vi "Device VI 1.2.vi"() -> ()   [LabVIEW 2017]
uses:
  <vilib>/Utility/error.llb/DialogType.ctl
  <vilib>/DAQmx/read.llb/DAQmx Read (Analog 1D Wfm NChan NSamp).vi
  <vilib>/DAQmx/create/channels.llb/DAQmx Create Channel (AI-Force-Bridge-Two-Point-Linear).vi
  <vilib>/DAQmx/configure/timing.llb/DAQmx Timing (Sample Clock).vi
  <vilib>/DAQmx/configure/trigger.llb/DAQmx Start Trigger (Digital Edge).vi
  <vilib>/DAQmx/configure/trigger.llb/DAQmx Start Trigger (Analog Edge).vi
  <vilib>/DAQmx/miscellaneous.llb/DAQmx Fill In Error Info.vi
  <resource>/objmgr/daqmx.rc
panel:
  in  "Filename":path=path "C:/Users/Julio/Desktop/Device Data/Test.xlsx"
  in  "Maximum Force":dbl=100.0
  in  "Minimum Force":dbl=-100.0
  in  "Units (Force)":i32(ring)=15875 items=["Newtons"=15875, "Pounds"=15876, "kgf"=15877, "From Custom Scale"=10065]
  in  "Trigger Type":T1(tab)
  in  "Digital Start Trigger Edge":i32(ring)=10280 caption="Edge" items=["Rising"=10280, "Falling"=10171]
  in  "Digital Start Trigger Source":tag="OnboardClock" caption="Source"
  in  "Digital Pause Trigger Pause When":i32(ring)=10192 caption="Pause When" items=["High"=10192, "Low"=10214]
  in  "Digital Pause Trigger Source":tag="/Dev1/PFI0" caption="Source"
  in  "Analog Start Trigger Level":dbl caption="Level" format="%0.2f"
  in  "Analog Start Trigger Hysteresis":dbl caption="Hysteresis" format="%.2f"
  in  "Analog Start Trigger Slope":i32(ring)=10280 caption="Slope" items=["Rising"=10280, "Falling"=10171]
  in  "Analog Start Trigger Source":string="APFI0" caption="Source"
  in  "Analog Pause Trigger Source":string="APFI0" caption="Source"
  in  "Analog Pause Trigger Pause When":i32(ring)=10093 caption="Pause When" items=["Above Level"=10093, "Below Level"=10107]
  in  "Analog Pause Trigger Level":dbl caption="Level" format="%.2f"
  in  "Bridge Information":T2={"Bridge Configuration"=10182, "Excitation Source"=10200, "Excitation Value"=2.5, "Nominal Resistance"=350.0} {"Excitation Source" items=["Internal"=10200, "External"=10167, "None"=10230]; "Bridge Configuration" items=["Full Bridge"=10182, "Half Bridge"=10187, "Quarter Bridge"=10270, "No Bridge"=10228]}
  in  "Physical Channel":tag="cDAQ2Mod1/ai0:cDAQ2Mod1/ai1"
  in  "Sample Rate":dbl=100.0
  in  "Samples per Loop":i32=100
  in  "Stop":bool
  out "Waveform Chart":waveform(dbl)[](graph)=[{"t0"=timestamp(3612197930.5365286 s since 1904-01-01), "dt"=0.01, "Y"=[-0.00735334478104631, -0.00735334478104631, -0.00735334478104631, -0.00735334478104631, -0.00735334478104631, -0.00735334478104631, -0.00735334478104631, -0.00735334478104631, -0.00735334478104631, -0.00735334478104631, -0.00735334478104631, -0.00735334478104631, -0.00735334478104631, -0.00735334478104631, -0.00735334478104631, -0.00735334478104631, -0.00735334478104631, -0.00735334478104631, -0.00735334478104631, -0.00735334478104631, -0.00735334478104631, -0.00735334478104631, -0.00735334478104631, -0.00735334478104631, -0.00735334478104631, -0.00735334478104631, -0.00735334478104631, -0.00735334478104631, -0.00735334478104631, -0.00735334478104631, -0.00735334478104631, -0.00735334478104631, -0.00735334478104631, -0.00735334478104631, -0.00735334478104631, -0.00735334478104631, -0.00735334478104631, -0.00735334478104631, -0.00735334478104631, -0.00735334478104631, -0.00735334478104631, -0.00735334478104631, -0.00735334478104631, -0.00735334478104631, -0.00735334478104631, -0.00735334478104631, -0.00735334478104631, -0.00735334478104631, -0.00735334478104631, -0.00735334478104631, -0.016674486052795045, -0.016674486052795045, -0.016674486052795045, -0.016674486052795045, -0.016674486052795045, -0.016674486052795045, -0.016674486052795045, -0.016674486052795045, -0.016674486052795045, -0.016674486052795045, -0.016674486052795045, -0.016674486052795045, -0.016674486052795045, -0.016674486052795045, -0.016674486052795045, -0.016674486052795045, -0.016674486052795045, -0.016674486052795045, -0.016674486052795045, -0.016674486052795045, -0.016674486052795045, -0.016674486052795045, -0.016674486052795045, -0.016674486052795045, -0.016674486052795045, -0.016674486052795045, -0.016674486052795045, -0.016674486052795045, -0.016674486052795045, -0.016674486052795045, -0.016674486052795045, -0.016674486052795045, -0.016674486052795045, -0.016674486052795045, -0.016674486052795045, -0.016674486052795045, -0.016674486052795045, -0.016674486052795045, -0.016674486052795045, -0.016674486052795045, -0.016674486052795045, -0.016674486052795045, -0.016674486052795045, -0.016674486052795045, -0.016674486052795045, -0.016674486052795045, -0.016674486052795045, -0.016674486052795045, -0.016674486052795045, -0.016674486052795045], "attributes"=variant("NI_ChannelName"=variant(string "cDAQ2Mod1/ai0"), "NI_UnitDescription"=variant(string "Newtons"))}, {"t0"=timestamp(3612197930.5365286 s since 1904-01-01), "dt"=0.01, "Y"=[0.0030034788542301913, 0.0030034788542301913, 0.0030034788542301913, 0.0030034788542301913, 0.0030034788542301913, 0.0030034788542301913, 0.0030034788542301913, 0.0030034788542301913, 0.0030034788542301913, 0.0030034788542301913, 0.0030034788542301913, 0.0030034788542301913, 0.0030034788542301913, 0.0030034788542301913, 0.0030034788542301913, 0.0030034788542301913, 0.0030034788542301913, 0.0030034788542301913, 0.0030034788542301913, 0.0030034788542301913, 0.0030034788542301913, 0.0030034788542301913, 0.0030034788542301913, 0.0030034788542301913, 0.0030034788542301913, 0.0030034788542301913, 0.0030034788542301913, 0.0030034788542301913, 0.0030034788542301913, 0.0030034788542301913, 0.0030034788542301913, 0.0030034788542301913, 0.0030034788542301913, 0.0030034788542301913, 0.0030034788542301913, 0.0030034788542301913, 0.0030034788542301913, 0.0030034788542301913, 0.0030034788542301913, 0.0030034788542301913, 0.0030034788542301913, 0.0030034788542301913, 0.0030034788542301913, 0.0030034788542301913, 0.0030034788542301913, 0.0030034788542301913, 0.0030034788542301913, 0.0030034788542301913, 0.0030034788542301913, 0.0030034788542301913, 0.00963184598080707, 0.00963184598080707, 0.00963184598080707, 0.00963184598080707, 0.00963184598080707, 0.00963184598080707, 0.00963184598080707, 0.00963184598080707, 0.00963184598080707, 0.00963184598080707, 0.00963184598080707, 0.00963184598080707, 0.00963184598080707, 0.00963184598080707, 0.00963184598080707, 0.00963184598080707, 0.00963184598080707, 0.00963184598080707, 0.00963184598080707, 0.00963184598080707, 0.00963184598080707, 0.00963184598080707, 0.00963184598080707, 0.00963184598080707, 0.00963184598080707, 0.00963184598080707, 0.00963184598080707, 0.00963184598080707, 0.00963184598080707, 0.00963184598080707, 0.00963184598080707, 0.00963184598080707, 0.00963184598080707, 0.00963184598080707, 0.00963184598080707, 0.00963184598080707, 0.00963184598080707, 0.00963184598080707, 0.00963184598080707, 0.00963184598080707, 0.00963184598080707, 0.00963184598080707, 0.00963184598080707, 0.00963184598080707, 0.00963184598080707, 0.00963184598080707, 0.00963184598080707, 0.00963184598080707, 0.00963184598080707, 0.00963184598080707], "attributes"=variant("NI_ChannelName"=variant(string "cDAQ2Mod1/ai1"), "NI_UnitDescription"=variant(string "Newtons"))}]
  # "Data"
  # "Settings"
  # "Trigger"
  # "This trigger type is not supported in continuous sample timing. \n\nRefer to your device documentation for more information on which triggers are supported."
  # "This trigger type is not supported in continuous sample timing. \n\nRefer to your device documentation for more information on which triggers are supported."
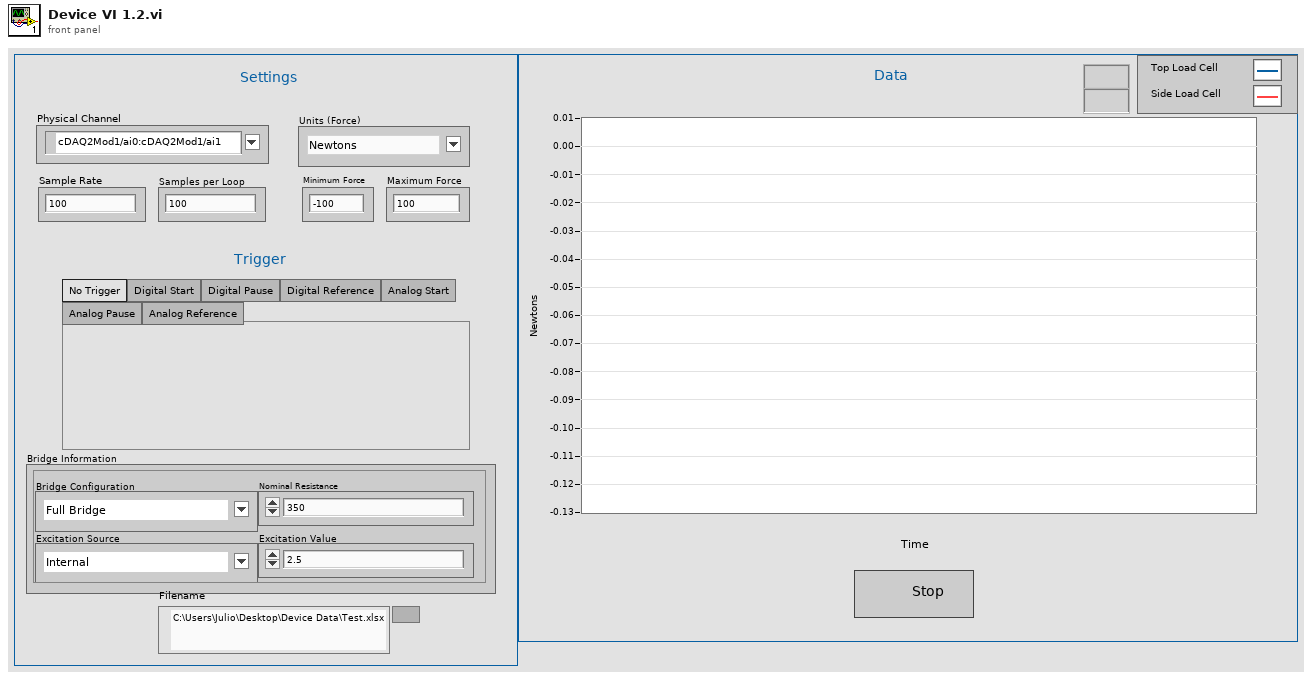
[diagram p1: front panel]
types:
  T1 = enum32{"No Trigger", "Digital Start", "Digital Pause", "Digital Reference", "Analog Start", "Analog Pause", "Analog Reference"}
  T2 = cluster{"Bridge Configuration":i32, "Excitation Source":i32, "Excitation Value":dbl, "Nominal Resistance":dbl}
  T3 = typedef "DialogType.ctl" = u16
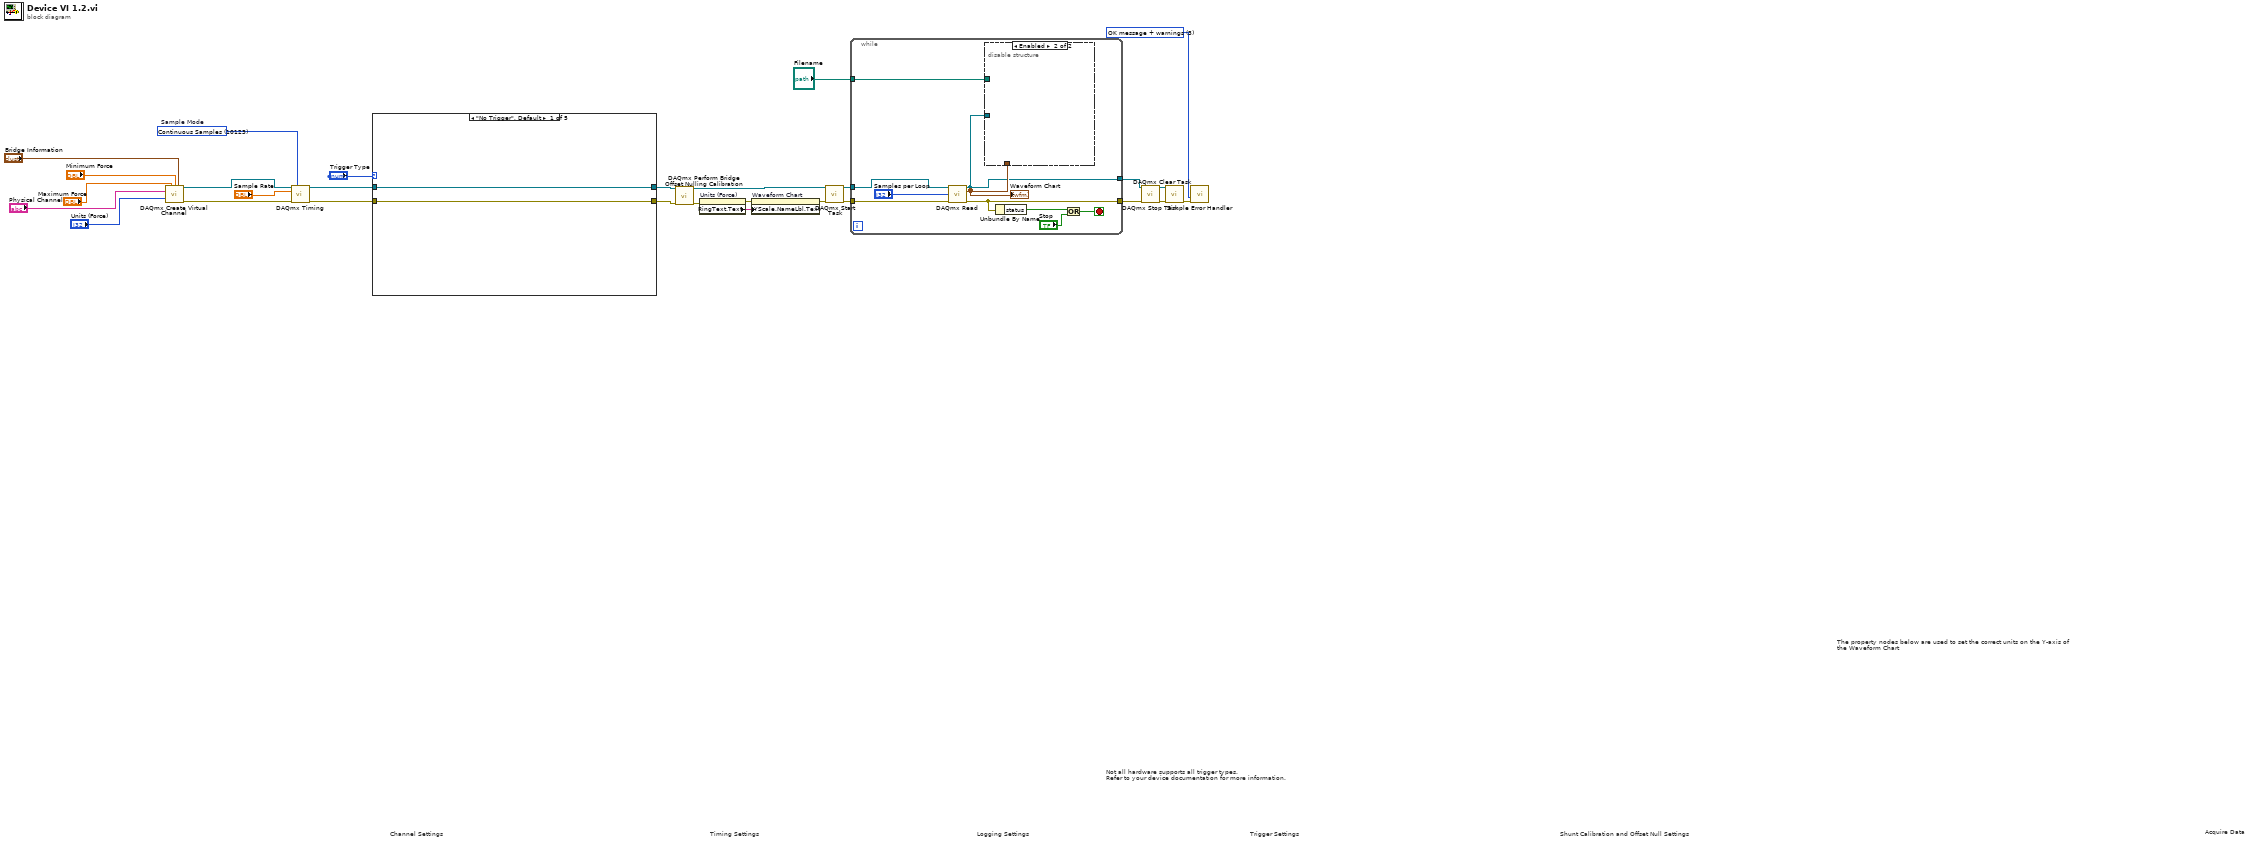
[diagram p0: block diagram]
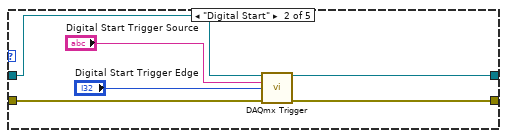
[diagram p2: hidden frame]
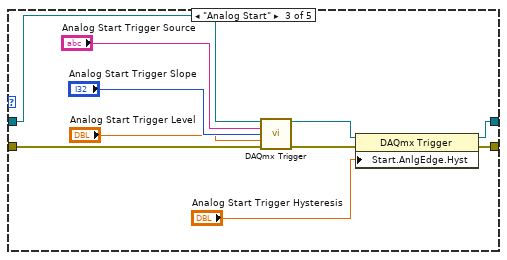
[diagram p3: hidden frame]
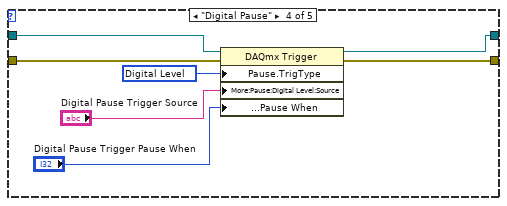
[diagram p4: hidden frame]
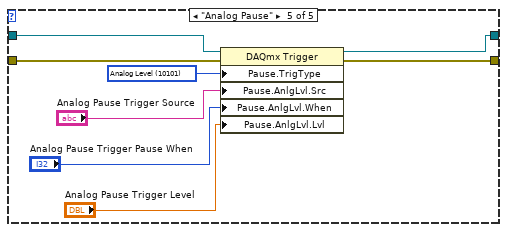
[diagram p5: hidden frame]
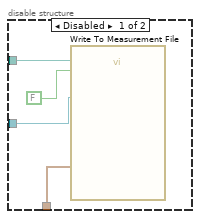
[diagram p6: hidden frame]
diagram:
  w14 = T3 3 items=["no dialog", "OK message", "continue or stop message", "OK message + warnings", "continue/stop + warnings"] ("type of dialog (OK msg:1)")
  w28 = 10123 items=["Finite Samples"=10178, "Continuous Samples"=10123, "Hardware Timed Single Point"=12522]  # Sample Mode
  # "Trigger Settings"
  # "Not all hardware supports all trigger types.\nRefer to your device documentation for more information."
  # "Logging Settings"
  # "The property nodes below are used to set the correct units on the Y-axis of the Waveform Chart"
  # "Acquire Data"
  # "Shunt Calibration and Offset Null Settings"
  # "Timing Settings"
  # "Channel Settings"
  n1 = call-poly <vilib>:"DAQmx Create Virtual Channel.vi"("maximum value"="Maximum Force", "minimum value"="Minimum Force", "bridge information"="Bridge Information", "physical channels"="Physical Channel", "units"="Units (Force)") -> ("task out"=w26:refnum<k21>, "error out"=w27:errorcluster)  [unwired: 9 in]
  n2 = call-poly <vilib>:"DAQmx Timing.vi"("task/channels in"=w26, "sample mode"=w28, "rate"="Sample Rate", "error in"=w27) -> ("task out"=w7:refnum<k21>, "error out"=w6:errorcluster)  [unwired: 10 in]
  n3 = case shown="\"No Trigger\", Default" "Trigger Type" {
    tunnel: w7 -> [w30 w36 w46 w53 w61]
    tunnel: w6 -> [w29 w35 w45 w50 w58]
    tunnel: [w30 w34 w43 w52 w60] -> w11
    tunnel: [w29 w33 w42 w51 w59] -> w12
    frame "No Trigger", Default {
    }
    frame "Digital Start" {
      n4 = call-poly <vilib>:"DAQmx Trigger.vi"("task/channels in"=w36, "source"="Digital Start Trigger Source", "edge"="Digital Start Trigger Edge", "error in"=w35) -> ("task out"=w34:refnum<k21>, "error out"=w33:errorcluster)  [unwired: 10 in]
    }
    frame "Analog Start" {
      n5 = call-poly <vilib>:"DAQmx Trigger.vi"("task/channels in"=w46, "source"="Analog Start Trigger Source", "slope"="Analog Start Trigger Slope", "level"="Analog Start Trigger Level", "error in"=w45) -> ("task out"=w41:refnum<k21>, "error out"=w40:errorcluster)  [unwired: 9 in]
      n6 = property class="DAQmx Trigger"(reference=w41, error in=w40, "Start.AnlgEdge.Hyst"="Analog Start Trigger Hysteresis") -> (reference out=w43:refnum<k21>, error out=w42:errorcluster)
    }
    frame "Digital Pause" {
      w49 = 10152 items=["Analog Level"=10101, "Analog Window"=10103, "Digital Level"=10152, "Digital Pattern"=10398, "None"=10230] ("Pause.TrigType")
      n7 = property class="DAQmx Trigger"(reference=w53, error in=w50, "Pause.TrigType"=w49, "More:Pause:Digital Level:Source"="Digital Pause Trigger Source", "More:Pause:Digital Level:Pause When"="Digital Pause Trigger Pause When") -> (reference out=w52:refnum<k21>, error out=w51:errorcluster)
    }
    frame "Analog Pause" {
      w57 = 10101 items=["Analog Level"=10101, "Analog Window"=10103, "Digital Level"=10152, "Digital Pattern"=10398, "None"=10230] ("Pause.TrigType")
      n8 = property class="DAQmx Trigger"(reference=w61, error in=w58, "Pause.TrigType"=w57, "Pause.AnlgLvl.Src"="Analog Pause Trigger Source", "Pause.AnlgLvl.When"="Analog Pause Trigger Pause When", "Pause.AnlgLvl.Lvl"="Analog Pause Trigger Level") -> (reference out=w60:refnum<k21>, error out=w59:errorcluster)
    }
  }
  n9 = call <vilib>:"DAQmx Perform Bridge Offset Nulling Calibration.vi"("task/channels in"=w11, "error in"=w12) -> ("task out"=w3:refnum<k21>, "error out"=w2:errorcluster)  [unwired: 12 in]
  n10 = property on="Units (Force)" class="Ring (strict)"(error in=w2) -> (error out=w5:errorcluster, "RingText.Text"=w4:string)  [unwired: 1 in, 1 out]
  n11 = property on="Waveform Chart" class="WFChart (strict)"(error in=w5, "YScale.NameLbl.Text"=w4) -> (error out=w20:errorcluster)  [unwired: 1 in, 1 out]
  n12 = call <vilib>:"DAQmx Start Task.vi"("task/channels in"=w3, "error in"=w20) -> ("task out"=w25:refnum<k21>, "error out"=w24:errorcluster)  [unwired: 12 in]
  n13 = while {
    tunnel: w25 -> [w71]
    tunnel: w24 -> [w70]
    tunnel: [w68] -> w17
    tunnel: [w63] -> w18
    tunnel: "Filename" -> [w62]
    stop <- w69 stop-if-true
    n14 = call-poly <vilib>:"DAQmx Read.vi"("task/channels in"=w71, "number of samples per channel"="Samples per Loop", "error in"=w70) -> ("task out"=w63:refnum<k21>, "data"=w64:waveform(dbl)[], "error out"=w68:errorcluster)  [unwired: 10 in]
    "Waveform Chart" <- w64
    n15 = disable-structure shown="Enabled" {
      disable-tunnel: w64 -> [w74 _]
      disable-tunnel: w63 -> [w73 _]
      disable-tunnel: w62 -> [w72 _]
      frame Disabled {
        n16 = call "Write To Measurement File"("Signals"=w74, "Enable"=FALSE, "Filename"=w72, "DAQmx Task"=w73) -> ()  [unwired: 13 in, 3 out]
      }
      frame Enabled {
      }
    }
    n17 = Unbundle By Name(w68) -> ("status"=w67:bool)
    n18 = Or(x=w67, y="Stop") -> (x .or. y?=w69:bool)
  }
  n19 = call <vilib>:"DAQmx Stop Task.vi"("task/channels in"=w18, "error in"=w17) -> ("task out"=w16:refnum<k21>, "error out"=w15:errorcluster)  [unwired: 12 in]
  n20 = call <vilib>:"DAQmx Clear Task.vi"("task in"=w16, "error in"=w15) -> ("error out"=w23:errorcluster)  [unwired: 13 in]
  n21 = call <vilib>:"Simple Error Handler.vi"("type of dialog (OK msg:1)"=w14, "error in (no error)"=w23) -> ()  [unwired: 3 in, 5 out]
